vi "Serial Number Query.vi"(8 "error in":errorcluster, 11 "VISA resource name":refnum<visa-resource-name>) -> (0 "error out":errorcluster, 2 "Serial Number":string, 3 "VISA resource name out":refnum<visa-resource-name>)   [LabVIEW 2011, in "DMM4.lvlib"]
uses:
  <instrlib>/DMM4/DMM4.lvlib
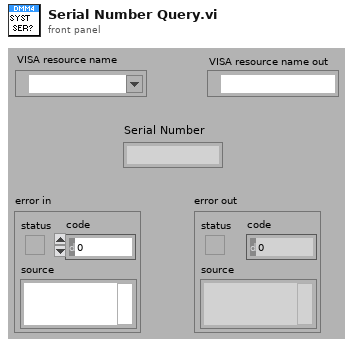
[diagram p1: front panel]
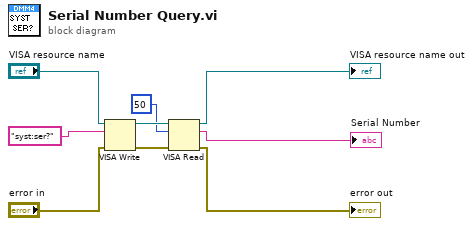
[diagram p0: block diagram]
diagram:
  n1 = VISA Write(VISA resource name="VISA resource name", write buffer="syst:ser?", error in (no error)="error in") -> (VISA resource name out=w6:refnum<visa-resource-name>, error out=w5:errorcluster)  [unwired: 1 out]
  n2 = VISA Read(VISA resource name=w6, byte count=u32 50, error in (no error)=w5) -> (VISA resource name out=→"VISA resource name out":refnum<visa-resource-name>, read buffer=→"Serial Number":string, error out=→"error out":errorcluster)  [unwired: 1 out]
